vi "Periodic Tasks.vi"(8 "error in":errorcluster) -> ()   [LabVIEW 2018]
doc: "This VI runs in parallel to other tasks. It can contain as many user-defined periodic loops as you need. These can carry out PID or other sorts of timed response."
uses:
  <vilib>/Rock Robotics/WPI/ThirdParty/Phoenix-LabVIEW/Pigeon IMU/CTRE_PigeonIMU_CalibrationMode.ctl
  <vilib>/Rock Robotics/WPI/ThirdParty/Phoenix-LabVIEW/Pigeon IMU/CTRE_PigeonIMU_PigeonState.ctl
  DriveLoopEnum.ctl
  <vilib>/Rock Robotics/WPI/Utilities/WPI_GetSetVariantRefNum.vi
  <vilib>/Rock Robotics/WPI/ThirdParty/Phoenix-LabVIEW/Motor Controller/Get/CTRE_Phoenix_MotorController_GetSelectedSensorData.vi
  <vilib>/Rock Robotics/WPI/ThirdParty/Phoenix-LabVIEW/Motor Controller/Get/CTRE_Phoenix_MotorController_GetVoltage.vi
  <vilib>/Utility/file.llb/Write Delimited Spreadsheet (DBL).vi
  <vilib>/Rock Robotics/WPI/ThirdParty/Phoenix-LabVIEW/Motor Controller/Get/CTRE_Phoenix_MotorController_GetClosedLoopData.vi
  <vilib>/Rock Robotics/WPI/ThirdParty/Phoenix-LabVIEW/Pigeon IMU/CTRE_PigeonIMU_GetTempStateUpTime.vi
  <vilib>/Rock Robotics/WPI/ThirdParty/Phoenix-LabVIEW/Pigeon IMU/CTRE_PigeonIMU_GetFusedHeading.vi
panel:
  out "Velocity":T1(graph)
  out "Error":cluster{"Closed-loop Error":i32, dbl}(graph)
  in  "D":dbl
  in  "I":dbl
  in  "P":dbl
  in  "Percent Max Speed":dbl
  in  "LowMaxSpeed":i32=7695
  out "Temp/State/UpTime":T4={"CurrentMode"=0, "LastCalError"=0, "CalBooting?"=FALSE, "PigeonState"=enum."Ready", "UpTime"=255, "Temp. (C)"=34.76953125, "Temp Compensation Event Count"=0, "No Motion Event Count"=0} {"CurrentMode" items=["BootTareGryoAccel"=0, "Temperature"=1, "Magnetometer12Pt"=2, "Magnetometer360"=3, "Accelerometer"=5]}
  out "Fused Heading":T5={"Heading"=373.0078125, "Valid?"=FALSE, "Fusing?"=FALSE}
  out "Right Position (Raw Sensor Units)":i32=1024961
  out "Left Position (Raw Sensor Units)":i32=868111
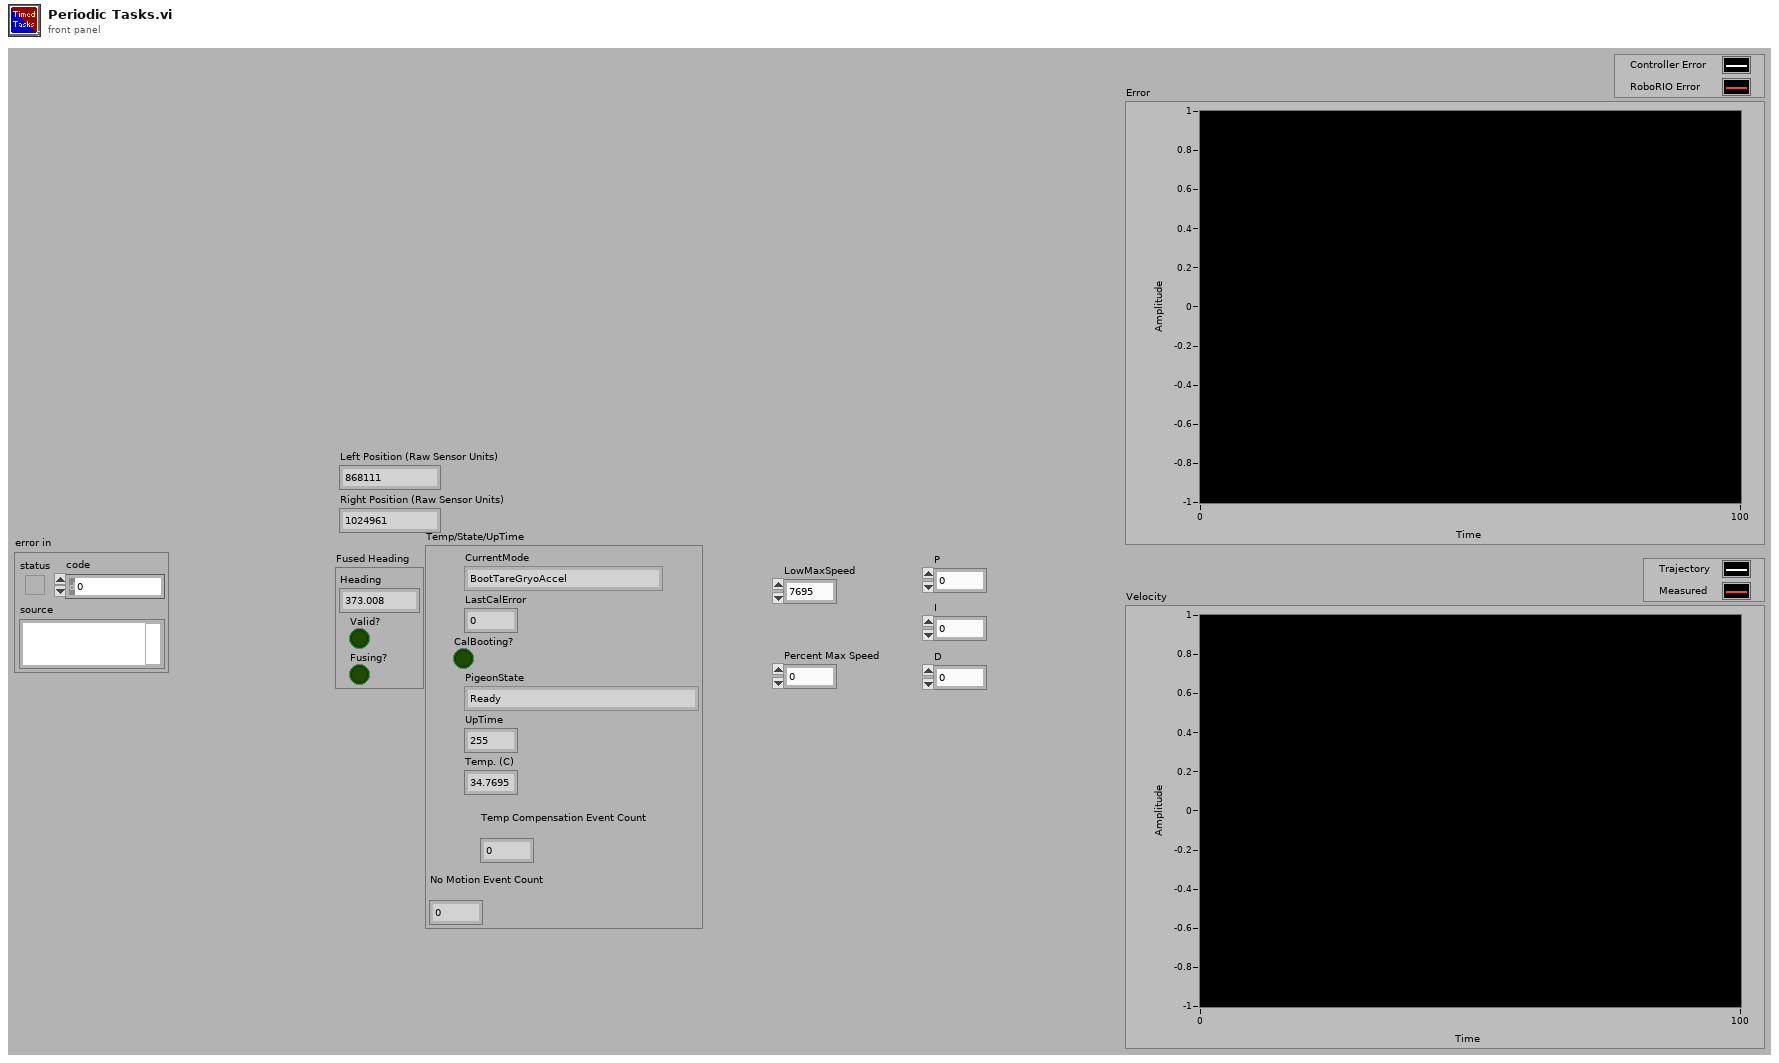
[diagram p1: front panel]
types:
  T1 = cluster{"Closed-loop Target":dbl, "Velocity (Raw Sensor Units per 100 ms)":i32}
  T2 = typedef "CTRE_PigeonIMU_CalibrationMode.ctl" = u16
  T3 = typedef "CTRE_PigeonIMU_PigeonState.ctl" = enum16{"NoComm", "Initializing", "Ready", "UserCalibration"}
  T4 = cluster{"CurrentMode":T2, "LastCalError":i32, "CalBooting?":bool, "PigeonState":T3, "UpTime":u32, "Temp. (C)":dbl, "Temp Compensation Event Count":u32, "No Motion Event Count":u32}
  T5 = cluster{"Heading":dbl, "Valid?":bool, "Fusing?":bool}
  T6 = typedef "WPI_JoystickDevRef.ctl" = cluster{"Device":T7}
  T7 = typedef "WPI_JoystickDeviceEnum.ctl" = enum16{"USB 0", "USB 1", "USB 2", "USB 3", "USB 4", "USB 5"}
  T8 = typedef "WPI_MotorControlDeviceRef.ctl" = cluster{"DeviceStatus":errorcluster, "Type":T9, "PWM":cluster{"PWM Channel":T10, "DeadBand":T11}, "CAN":cluster{"Device Number":u8, "SetOutput VI Ref":variant, "GetOutput VI Ref":variant, "Enable VI Ref":variant, "Disable VI Ref":variant, "Data":variant}, "Invert":bool, "DIO PWM":cluster{"PWM \"Enable\" Channel":T10, "DIOChannel":T12, "PWM Rate":dbl}}
  T9 = typedef "WPI_MotorControlType.ctl" = enum16{"PWM", "CAN", "DIO PWM"}
  T10 = typedef "FPGA_DIOPWMChannel.ctl" = enum8{"PWM 0", "PWM 1", "PWM 2", "PWM 3", "PWM 4", "PWM 5", "PWM 6", "PWM 7", "PWM 8", "PWM 9", "PWM MXP 0", "PWM MXP 1", "PWM MXP 2", "PWM MXP 3", "PWM MXP 4", "PWM MXP 5", "PWM MXP 6", "PWM MXP 7", "PWM MXP 8", "PWM MXP 9", "Invalid"}
  T11 = typedef "WPI_PWMDeadband.ctl" = cluster{"Name":string, "maxPositivePwm":i32, "minPositivePwm":i32, "centerPwm":i32, "maxNegativePwm":i32, "minNegativePwm":i32, "angularRange":u16}
  T12 = typedef "FPGA_DIOChannel.ctl" = enum8{"DIO 0", "DIO 1", "DIO 2", "DIO 3", "DIO 4", "DIO 5", "DIO 6", "DIO 7", "DIO 8", "DIO 9", "DIO MXP 0", "DIO MXP 1", "DIO MXP 2", "DIO MXP 3", "DIO MXP 4", "DIO MXP 5", "DIO MXP 6", "DIO MXP 7", "DIO MXP 8", "DIO MXP 9", "DIO MXP 10", "DIO MXP 11", "DIO MXP 12", "DIO MXP 13", "DIO MXP 14", "DIO MXP 15", "SPI Port CS1", "SPI Port CS2", "SPI Port CS3", "SPI Port MISO", "SPI Port MOSI", "Invalid"}
  T13 = typedef "DriveLoopEnum.ctl" = enum16{"Manual", "Velocity Control", "Motion Magic"}
  T14 = cluster{"Velocity (tick/100ms)":dbl, "Output Voltage":dbl, "Bus Voltage":dbl}
  T15 = typedef "CTRE_PigeonIMU_DeviceRef.ctl" = cluster{"DeviceStatus":errorcluster, "Device Number":u8, "Type":T16, "Device ID":u32, "Handle":u64, "UsageFrame":u32, "Library Path":path}
  T16 = typedef "CTRE_PigeonIMU_ConnectionType.ctl" = u32
  T17 = cluster{dbl, "Velocity (Raw Sensor Units per 100 ms)":i32}
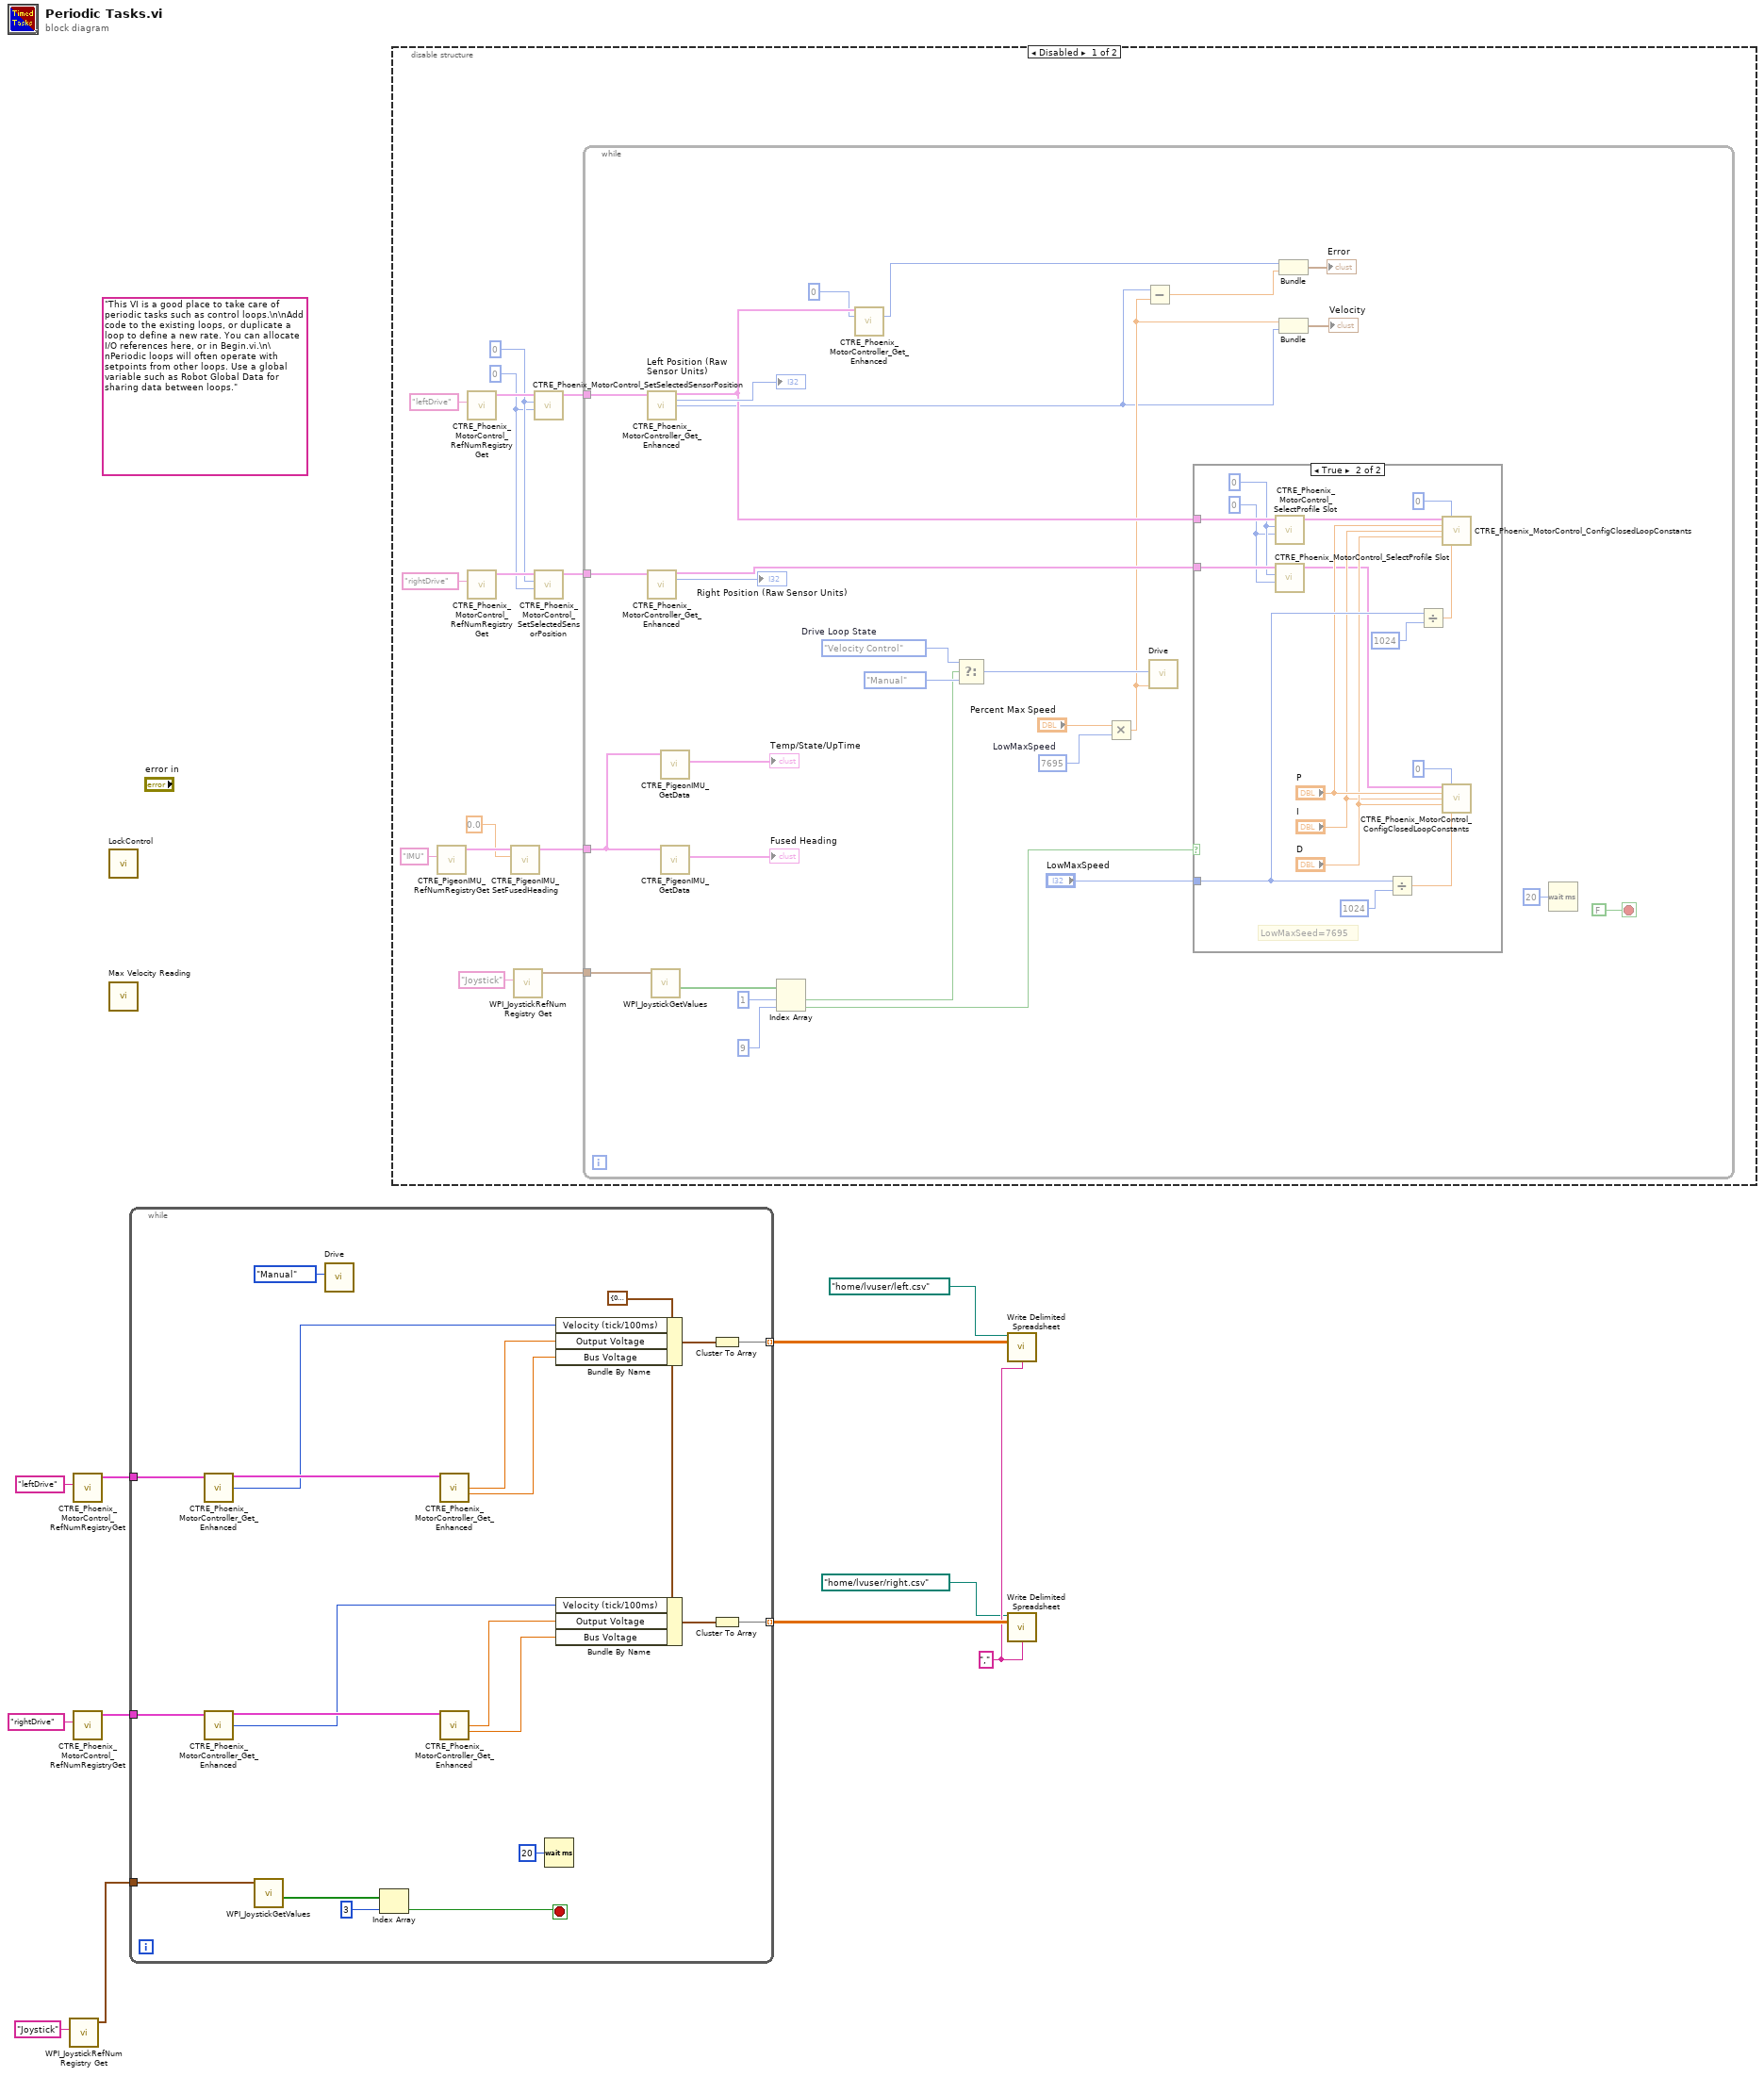
[diagram p0: block diagram]
diagram:
  w5 = "," ("delimiter (\\t)")
  (unwired) "This VI is a good place to take care of periodic tasks such as control loops.\n\nAdd code to the existing loops, or duplicate a loop to define a new rate. You can allocate I/O references here, or in Begin.vi.\n\nPeriodic loops will often operate with setpoints from other loops. Use a global variable such as Robot Global Data for sharing data between loops."
  n1 = call <vilib>:"WPI_JoystickRefNum Registry Get.vi"("refnum name"="Joystick") -> ("JoystickDevRef"=w1:T6)  [unwired: 9 in, 1 out]
  n2 = call <vilib>:"CTRE_Phoenix_MotorControl_RefNumRegistryGet.vi"("refnum name"="leftDrive") -> ("PhoenixMotorControlDevRef"=w9:T8)  [unwired: 9 in, 1 out]
  n3 = call <vilib>:"CTRE_Phoenix_MotorControl_RefNumRegistryGet.vi"("refnum name"="rightDrive") -> ("PhoenixMotorControlDevRef"=w8:T8)  [unwired: 9 in, 1 out]
  n4 = call "LockControl.vi"() -> ()  [unwired: 12 in]
  n5 = call "Max Velocity Reading.vi"() -> ()  [unwired: 12 in]
  n6 = while {
    tunnel: w9 -> [w31]
    tunnel: w8 -> [w30]
    tunnel: [w19] -> w7 mode=indexing
    tunnel: [w17] -> w6 mode=indexing
    tunnel: w1 -> [w14]
    stop <- w13 stop-if-true
    w27 = T14 {"Velocity (tick/100ms)"=0.0, "Output Voltage"=0.0, "Bus Voltage"=0.0} ("Data Point")
    n7 = call-poly <vilib>:"CTRE_Phoenix_MotorController_Get_Enhanced.vi"("PhoenixMotorControlDevRef"=w31) -> ("PhoenixMotorControlDevRef"=w28:T8, "Velocity (Raw Sensor Units per 100 ms)"=w24:i32)  [unwired: 11 in, 2 out]
    n8 = call-poly <vilib>:"CTRE_Phoenix_MotorController_Get_Enhanced.vi"("PhoenixMotorControlDevRef"=w30) -> ("PhoenixMotorControlDevRef"=w29:T8, "Velocity (Raw Sensor Units per 100 ms)"=w23:i32)  [unwired: 11 in, 2 out]
    n9 = call <vilib>:"WPI_JoystickGetValues.vi"("JoystickDevRef"=w14) -> ("Buttons"=w16:bool[])  [unwired: 6 in, 4 out]
    n10 = call "Drive.vi"("Drive Loop State"=DriveLoopEnum."Manual") -> ()  [unwired: 11 in]
    n11 = Index Array(array=w16, index=3) -> (element=w13:bool)
    n12 = call-poly <vilib>:"CTRE_Phoenix_MotorController_Get_Enhanced.vi"("PhoenixMotorControlDevRef"=w28) -> ("Output Voltage"=w26:dbl, "Bus Voltage"=w25:dbl)  [unwired: 10 in, 3 out]
    n13 = call-poly <vilib>:"CTRE_Phoenix_MotorController_Get_Enhanced.vi"("PhoenixMotorControlDevRef"=w29) -> ("Output Voltage"=w22:dbl, "Bus Voltage"=w21:dbl)  [unwired: 10 in, 3 out]
    n14 = Wait (ms)(milliseconds to wait=u32 20) -> ()  [unwired: 1 out]
    n15 = Bundle By Name(cluster=w27, "Velocity (tick/100ms)"=w24, "Output Voltage"=w26, "Bus Voltage"=w25) -> (w20:T14)
    n16 = Bundle By Name(cluster=w27, "Velocity (tick/100ms)"=w23, "Output Voltage"=w22, "Bus Voltage"=w21) -> (w18:T14)
    n17 = Cluster To Array(cluster=w20) -> (array=w19:dbl[])
    n18 = Cluster To Array(cluster=w18) -> (array=w17:dbl[])
  }
  n19 = disable-structure shown="Disabled" {
    frame Disabled {
      w39 = u32 0 ("pidLoopIdx")
      w40 = 0 ("New Sensor Position")
      n20 = call <vilib>:"CTRE_PigeonIMU_RefNumRegistryGet.vi"("refnum name"="IMU") -> ("PigeonIMUDevRef"=w37:T15)  [unwired: 9 in, 1 out]
      n21 = call <vilib>:"CTRE_Phoenix_MotorControl_RefNumRegistryGet.vi"("refnum name"="leftDrive") -> ("PhoenixMotorControlDevRef"=w44:T8)  [unwired: 9 in, 1 out]
      n22 = call <vilib>:"CTRE_Phoenix_MotorControl_RefNumRegistryGet.vi"("refnum name"="rightDrive") -> ("PhoenixMotorControlDevRef"=w42:T8)  [unwired: 9 in, 1 out]
      n23 = call <vilib>:"CTRE_PigeonIMU_SetFusedHeading.vi"("Value"=0.0, "PigeonIMUDevRef 2"=w37) -> ("PigeonIMUDevRef"=w36:T15)  [unwired: 8 in, 1 out]
      n24 = call <vilib>:"WPI_JoystickRefNum Registry Get.vi"("refnum name"="Joystick") -> ("JoystickDevRef"=w33:T6)  [unwired: 9 in, 1 out]
      n25 = call <vilib>:"CTRE_Phoenix_MotorControl_SetSelectedSensorPosition.vi"("pidLoopIdx"=w39, "New Sensor Position"=w40, "PhoenixMotorControlDevRef"=w44) -> ("PhoenixMotorControlDevRef"=w43:T8)  [unwired: 7 in, 1 out]
      n26 = call <vilib>:"CTRE_Phoenix_MotorControl_SetSelectedSensorPosition.vi"("pidLoopIdx"=w39, "New Sensor Position"=w40, "PhoenixMotorControlDevRef"=w42) -> ("PhoenixMotorControlDevRef"=w41:T8)  [unwired: 7 in, 1 out]
      n27 = while {
        tunnel: w43 -> [w74]
        tunnel: w41 -> [w73]
        tunnel: w36 -> [w72]
        tunnel: w33 -> [w63]
        stop <- FALSE stop-if-true
        w65 = 7695  # LowMaxSpeed
        w67 = DriveLoopEnum."Velocity Control"  # Drive Loop State
        n28 = call-poly <vilib>:"CTRE_Phoenix_MotorController_Get_Enhanced.vi"("PhoenixMotorControlDevRef"=w74) -> ("PhoenixMotorControlDevRef"=w54:T8, "Position (Raw Sensor Units)"=→"Left Position (Raw Sensor Units)":i32, "Velocity (Raw Sensor Units per 100 ms)"=w50:i32)  [unwired: 11 in, 1 out]
        n29 = call-poly <vilib>:"CTRE_Phoenix_MotorController_Get_Enhanced.vi"("PhoenixMotorControlDevRef"=w73) -> ("PhoenixMotorControlDevRef"=w55:T8, "Position (Raw Sensor Units)"=→"Right Position (Raw Sensor Units)":i32)  [unwired: 11 in, 2 out]
        n30 = call <vilib>:"WPI_JoystickGetValues.vi"("JoystickDevRef"=w63) -> ("Buttons"=w62:bool[])  [unwired: 6 in, 4 out]
        n31 = call-poly <vilib>:"CTRE_PigeonIMU_GetData.vi"("PigeonIMUDevRef"=w72) -> ("Temp/State/UpTime"=→"Temp/State/UpTime":T4)  [unwired: 8 in, 2 out]
        n32 = call-poly <vilib>:"CTRE_PigeonIMU_GetData.vi"("PigeonIMUDevRef"=w72) -> ("Fused Heading"=→"Fused Heading":T5)  [unwired: 8 in, 2 out]
        n33 = Index Array(array=w62, index #1=1 ("index"), index #2=9 ("index")) -> (element #1=w58:bool, element #2=w61:bool)
        n34 = call-poly <vilib>:"CTRE_Phoenix_MotorController_Get_Enhanced.vi"("PhoenixMotorControlDevRef"=w54, "pidLoopIdx"=0) -> ("Closed-loop Error"=w47:i32)  [unwired: 8 in, 5 out]
        n35 = Select(t=w67, s=w58, f=DriveLoopEnum."Manual") -> (s? t:f=w60:T13)
        n36 = Multiply(x="Percent Max Speed", y=w65) -> (x*y=w51:dbl)
        n37 = Subtract(x=w50, y=w51) -> (x-y=w48:dbl)
        n38 = call "Drive.vi"("Velocity Setting"=w51, "Drive Loop State"=w60) -> ()  [unwired: 10 in]
        n39 = case shown="True" w61 {
          tunnel: "LowMaxSpeed" -> [_ w86]
          tunnel: w54 -> [_ w82]
          tunnel: w55 -> [_ w80]
          frame False {
          }
          frame True {
            w77 = 0 ("pidLoopIdx")
            w78 = 0 ("slotIdx")
            # "LowMaxSeed=7695"
            n40 = call <vilib>:"CTRE_Phoenix_MotorControl_SelectProfile Slot.vi"("pidLoopIdx"=w77, "slotIdx"=w78, "PhoenixMotorControlDevRef"=w82) -> ("PhoenixMotorControlDevRef"=w81:T8)  [unwired: 7 in, 1 out]
            n41 = call <vilib>:"CTRE_Phoenix_MotorControl_SelectProfile Slot.vi"("pidLoopIdx"=w77, "slotIdx"=w78, "PhoenixMotorControlDevRef"=w80) -> ("PhoenixMotorControlDevRef"=w79:T8)  [unwired: 7 in, 1 out]
            n42 = Divide(x=w86, y=1024) -> (x/y=w91:dbl)
            n43 = Divide(x=w86, y=1024) -> (x/y=w88:dbl)
            n44 = call <vilib>:"CTRE_Phoenix_MotorControl_ConfigClosedLoopConstants.vi"("PhoenixMotorControlDevRef"=w81, "slotIdx"=0, "P"="P", "I"="I", "D"="D", "F"=w88) -> ()  [unwired: 8 in, 2 out]
            n45 = call <vilib>:"CTRE_Phoenix_MotorControl_ConfigClosedLoopConstants.vi"("PhoenixMotorControlDevRef"=w79, "slotIdx"=0, "P"="P", "I"="I", "D"="D", "F"=w91) -> ()  [unwired: 8 in, 2 out]
          }
        }
        n46 = Bundle("Closed-loop Error"=w47, w48) -> (→"Error":cluster{"Closed-loop Error":i32, dbl})  [unwired: 1 in]
        n47 = Bundle(w51, "Velocity (Raw Sensor Units per 100 ms)"=w50) -> (→"Velocity":T17)  [unwired: 1 in]
        n48 = Wait (ms)(milliseconds to wait=u32 20) -> ()  [unwired: 1 out]
      }
    }
    frame Enabled {
    }
  }
  n49 = call-poly <vilib>:"Write Delimited Spreadsheet.vi"("file path (dialog if empty)"=path "/home/lvuser/left.csv", "2D data"=w7, "delimiter (\\t)"=w5) -> ()  [unwired: 11 in, 2 out]
  n50 = call-poly <vilib>:"Write Delimited Spreadsheet.vi"("file path (dialog if empty)"=path "/home/lvuser/right.csv", "2D data"=w6, "delimiter (\\t)"=w5) -> ()  [unwired: 11 in, 2 out]
